vi "Untitled 3.vi"() -> ()   [LabVIEW 2023]
uses:
  <vilib>/numeric/Random Number (Range) U64.vi
  <vilib>/numeric/sub_Random U32.vi
  <vilib>/Analysis/NI_AALPro.lvlib
panel:
  out "interpolation value":dbl format="%0.2f"
  out "XY Graph 3":cluster{dbl[], "Best Exponential Fit":dbl[]}(graph)
  out "XY Graph 2":cluster{dbl[], "Best Exponential Fit":dbl[]}(graph)
  out "Array":u64[](array[numeric])
  out "amplitude":dbl
  out "Best Exponential Fit":dbl[](array[numeric])
  out "XY Graph":cluster{dbl[], u64[]}(graph)
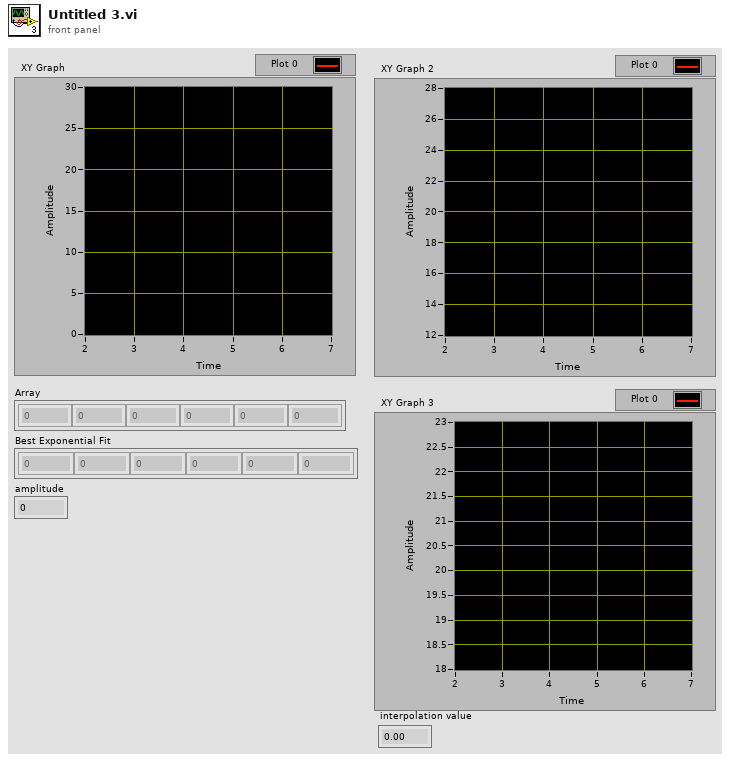
[diagram p1: front panel]
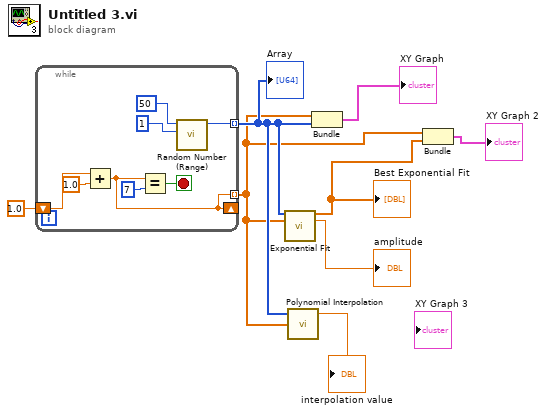
[diagram p0: block diagram]
diagram:
  n1 = while {
    tunnel: [w10] -> w2 mode=indexing
    tunnel: [w9] -> w3 mode=indexing
    shift-right: [w10] -> _
    shift-left: 1.0 ("y") -> [w11]
    stop <- w13 stop-if-true
    n2 = Add(x=w11, y=1.0) -> (x+y=w10:dbl)
    n3 = Equal?(x=w10, y=u64 7) -> (x = y?=w13:bool)
    n4 = call-poly <vilib>:"Random Number (Range).vi"("lower bound (0)"=u64 1, "upper bound (100)"=u64 50) -> ("number"=w9:u64)  [unwired: 9 in]
  }
  "Array" <- w3
  n5 = call <vilib>:"Exponential Fit.vi"("Y"=w3, "X"=w2) -> ("Best Exponential Fit"=w5:dbl[], "amplitude"=→"amplitude":dbl)  [unwired: 8 in, 4 out]
  "Best Exponential Fit" <- w5
  n6 = call <vilib>:"Polynomial Interpolation.vi"("X"=w2, "Y"=w3) -> ("interpolation value"=→"interpolation value":dbl)  [unwired: 1 in, 2 out]
  n7 = Bundle(w2, w3) -> (→"XY Graph":cluster{dbl[], u64[]})  [unwired: 1 in]
  n8 = Bundle(w2, "Best Exponential Fit"=w5) -> (→"XY Graph 2":cluster{dbl[], "Best Exponential Fit":dbl[]})  [unwired: 1 in]
